vi "tsdiag_can_create.vi"(8 "错误输入（无错误）":errorcluster, 10 "Cluster":T1, 11 "path":path) -> (0 "错误输出":errorcluster, 1 "pDiagModuleIndex":i32, 2 "Return Type":i32, 3 "path output":path)   [LabVIEW 2014]
doc: "Function Introduction :\nCreate CAN UDS diagnostic service\nCall location :\ninput parameter :\nPDiagModulus Index: Save the int pointer of the UDS module, which is used as a sentence by all diagnostic APIs\nhandle\nAChnIndex: Channel Index\nASupportFDCAN: Does it support FDCAN mode\nAMaxDLC: Maximum data length of canfd frame\nARequestID: request ID for UDS ARequestIDIsStad: whether the request ID is a standard ID AResponseID: response for UDS I AResponseIDIsStad: whether the response ID is a standard ID AFunctionID: UDS function ID AFunctionIDIsStad: whether the function ID is a standard ID\nReturn value :\n==0: Execution successful\nOther values: Query error code"
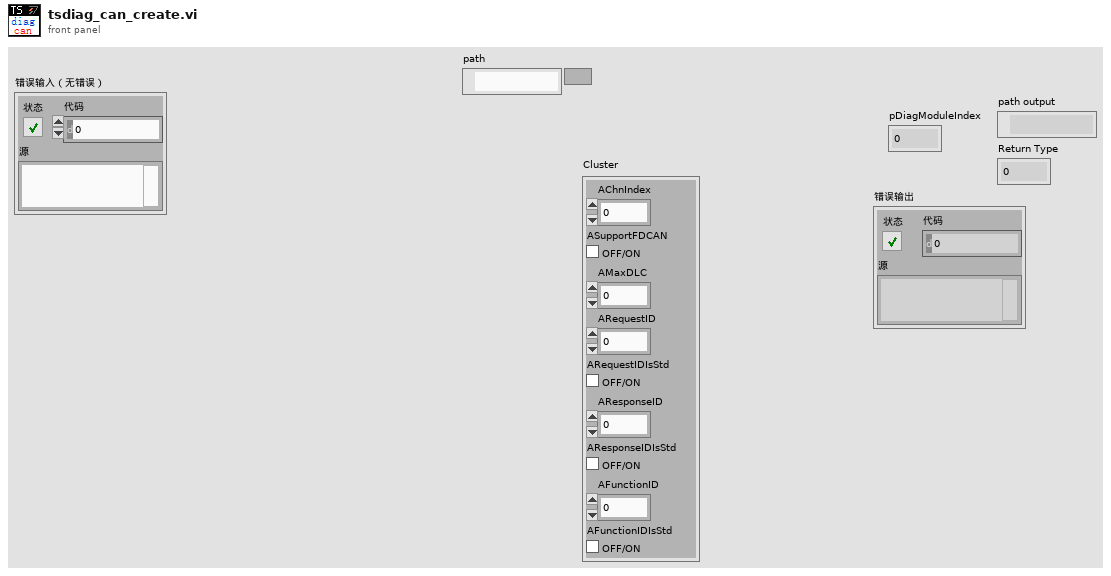
[diagram p1: front panel]
types:
  T1 = cluster{"AChnIndex":u32, "ASupportFDCAN":bool, "AMaxDLC":u16, "ARequestID":u32, "ARequestIDIsStd":bool, "AResponseID":u32, "AResponseIDIsStd":bool, "AFunctionID":u32, "AFunctionIDIsStd":bool}
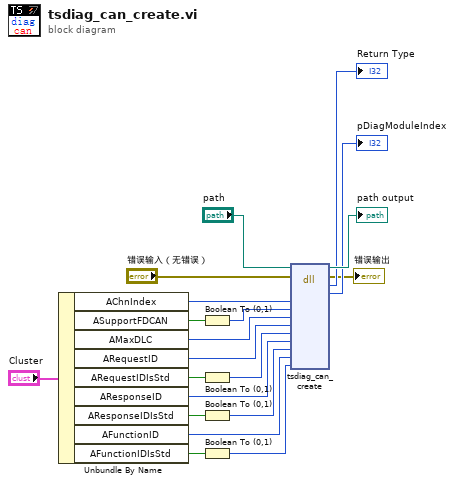
[diagram p0: block diagram]
diagram:
  n1 = Unbundle By Name("Cluster") -> ("AChnIndex"=w16:u32, "ASupportFDCAN"=w15:bool, "AMaxDLC"=w14:u16, "ARequestID"=w13:u32, "ARequestIDIsStd"=w12:bool, "AResponseID"=w1:u32, "AResponseIDIsStd"=w11:bool, "AFunctionID"=w10:u32, "AFunctionIDIsStd"=w9:bool)
  n2 = Boolean To (0,1)(Boolean=w15) -> (0, 1=w5:i16)
  n3 = Boolean To (0,1)(Boolean=w12) -> (0, 1=w4:i16)
  n4 = Boolean To (0,1)(Boolean=w11) -> (0, 1=w3:i16)
  n5 = Boolean To (0,1)(Boolean=w9) -> (0, 1=w2:i16)
  n6 = dll-call lib="C:/Users/XYY/Desktop/LabView Demo/TSCAN_LB2018_V1.3_20220301/Config/TSMaster.dll" fn="tsdiag_can_create"(path in="path", error in="错误输入（无错误）", "AChnIndex"=w16, "ASupportFDCAN"=w5, "AMaxDLC"=w14, "ARequestID"=w13, "ARequestIDIsStd"=w4, "AResponseID"=w1, "AResponseIDIsStd"=w3, "AFunctionID"=w10, "AFunctionIDIsStd"=w2) -> (path out=→"path output":path, error out=→"错误输出":errorcluster, "返回类型"=→"Return Type":i32, "pDiagModuleIndex"=→"pDiagModuleIndex":i32)  [unwired: 11 in]
